vi "VI Tree.vi"   [LabVIEW 2019, in "BK Precision 8500B Series.lvlib"]
doc: "This is the instrument driver for the BK Precision 8500B series DC electronic loads. The VI Tree displays all the user-callable VIs of the instrument driver in an organized table."
uses:
  <instrlib>/BK Precision 8500B Series/BK Precision 8500B Series.lvlib
panel:
  # "(c) 2019 B&K Precision Corporation.  ALL RIGHTS RESERVED."
  # "SEE DIAGRAM\nFOR VI TREE."
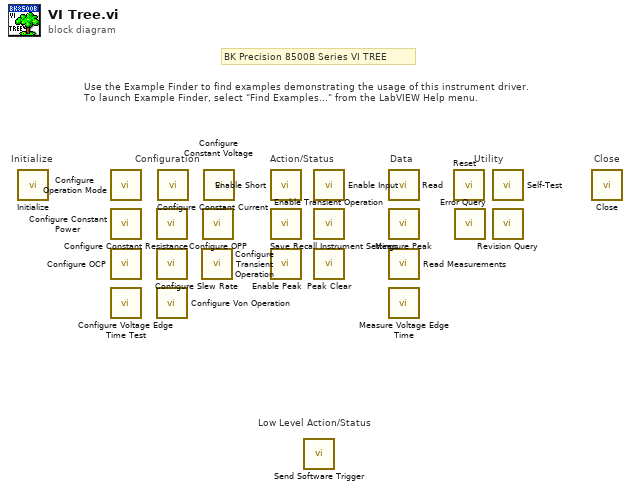
[diagram p0: block diagram]
diagram:
  # "Low Level Action/Status"
  # "BK Precision 8500B Series VI TREE"
  # "Use the Example Finder to find examples demonstrating the usage of this instrument driver.\nTo launch Example Finder, select \"Find Examples...\" from the LabVIEW Help menu."
  # "Configuration"
  # "Utility"
  # "Data"
  # "Action/Status"
  # "Close"
  # "Initialize"
  n1 = call <instrlib>:"Initialize.vi"() -> ()  [unwired: 10 in, 2 out]
  n2 = call <instrlib>:"Configure Operation Mode.vi"() -> ()  [unwired: 10 in, 2 out]
  n3 = call <instrlib>:"Configure Constant Power.vi"() -> ()  [unwired: 10 in, 2 out]
  n4 = call <instrlib>:"Configure OCP.vi"() -> ()  [unwired: 10 in, 2 out]
  n5 = call <instrlib>:"Configure Voltage Edge Time Test.vi"() -> ()  [unwired: 10 in, 2 out]
  n6 = call <instrlib>:"Configure Constant Resistance.vi"() -> ()  [unwired: 10 in, 2 out]
  n7 = call <instrlib>:"Configure Slew Rate.vi"() -> ()  [unwired: 10 in, 2 out]
  n8 = call <instrlib>:"Configure Von Operation.vi"() -> ()  [unwired: 10 in, 2 out]
  n9 = call <instrlib>:"Configure Constant Current.vi"() -> ()  [unwired: 10 in, 2 out]
  n10 = call <instrlib>:"Configure Transient Operation.vi"() -> ()  [unwired: 14 in, 2 out]
  n11 = call <instrlib>:"Configure OPP.vi"() -> ()  [unwired: 10 in, 2 out]
  n12 = call <instrlib>:"Configure Constant Voltage.vi"() -> ()  [unwired: 10 in, 2 out]
  n13 = call <instrlib>:"Enable Short.vi"() -> ()  [unwired: 10 in, 2 out]
  n14 = call <instrlib>:"Save Recall Instrument Settings.vi"() -> ()  [unwired: 10 in, 2 out]
  n15 = call <instrlib>:"Enable Peak.vi"() -> ()  [unwired: 10 in, 2 out]
  n16 = call <instrlib>:"Send Software Trigger.vi"() -> ()  [unwired: 10 in, 2 out]
  n17 = call <instrlib>:"Enable Input.vi"() -> ()  [unwired: 10 in, 2 out]
  n18 = call <instrlib>:"Enable Transient Operation.vi"() -> ()  [unwired: 10 in, 2 out]
  n19 = call <instrlib>:"Peak Clear.vi"() -> ()  [unwired: 10 in, 2 out]
  n20 = call <instrlib>:"Read.vi"() -> ()  [unwired: 8 in, 4 out]
  n21 = call <instrlib>:"Measure Peak.vi"() -> ()  [unwired: 6 in, 6 out]
  n22 = call <instrlib>:"Read Measurements.vi"() -> ()  [unwired: 8 in, 12 out]
  n23 = call <instrlib>:"Measure Voltage Edge Time.vi"() -> ()  [unwired: 8 in, 4 out]
  n24 = call <instrlib>:"Reset.vi"() -> ()  [unwired: 10 in, 2 out]
  n25 = call <instrlib>:"Error Query.vi"() -> ()  [unwired: 8 in, 4 out]
  n26 = call <instrlib>:"Self-Test.vi"() -> ()  [unwired: 8 in, 4 out]
  n27 = call <instrlib>:"Revision Query.vi"() -> ()  [unwired: 8 in, 4 out]
  n28 = call <instrlib>:"Close.vi"() -> ()  [unwired: 11 in, 1 out]
